vi "ClassAppData.Save.vi"(8 "error in (no error)":errorcluster, 11 "Class - App Data in":refnum<class "Class.AppData.lvclass">) -> (0 "error out":errorcluster, 3 "Class - App Data out":refnum<class "Class.AppData.lvclass">)   [LabVIEW 2024, in "EQMF.lvlib" / "Config Utils.lvlib" / "Class.AppData.lvclass"]
uses:
  Class.AppData.lvclass
  Class.AppData.lvclass/Class.AppData.ctl
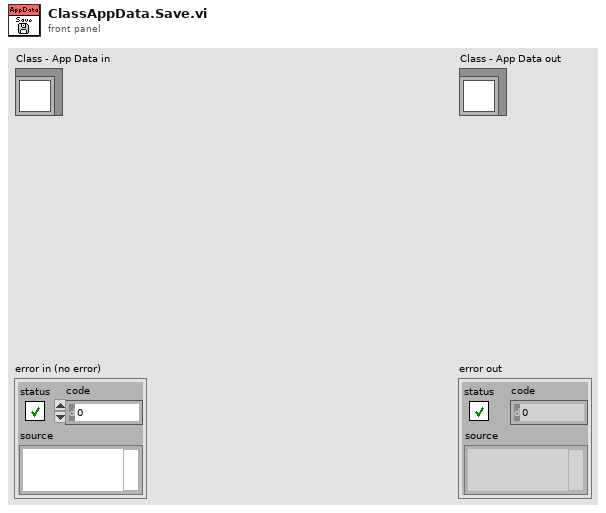
[diagram p1: front panel]
types:
  T1 = enum16{"open", "replace", "create", "open or create", "replace or create", "replace or create with confirmation"}
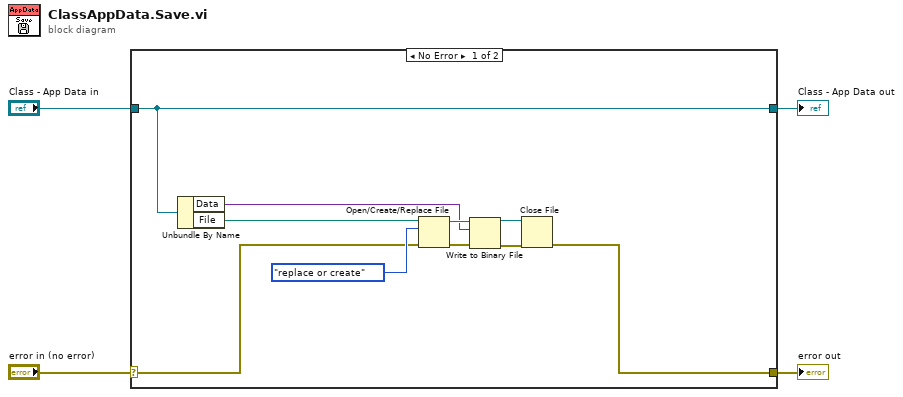
[diagram p0: block diagram]
diagram:
  n1 = case shown="No Error" "error in (no error)" {
    selector: "error in (no error)" -> [w6 w16]
    tunnel: [w5 w16] -> w3
    tunnel: [w14 w15] -> w1
    tunnel: "Class - App Data in" -> [w14 w15]
    frame No Error {
      n2 = Unbundle By Name(w14) -> ("Data"=w7:variant, "File"=w8:path)
      n3 = Open/Create/Replace File(file path (use dialog)=w8, error in=w6, operation (0:open)=T1."replace or create") -> (refnum out=w10:refnum<file>, error out=w11:errorcluster)  [unwired: 3 in, 1 out]
      n4 = Write to Binary File(file (use dialog)=w10, data=w7, error in=w11) -> (refnum out=w12:refnum<file>, error out=w13:errorcluster)  [unwired: 3 in, 1 out]
      n5 = Close File(refnum=w12, error in=w13) -> (error out=w5:errorcluster)  [unwired: 1 out]
    }
    frame Error {
    }
  }
  "error out" <- w3
  "Class - App Data out" <- w1
